vi "Amp_Lat_Finder.vi"(1 "ERP_vector":dbl[](array[numeric])) -> (0 "LDA_Parameter":dbl[][](array[numeric]))   [LabVIEW 2014]
uses:
  <vilib>/Analysis/baseanly.llb/Mean (DBL).vi
  <vilib>/Analysis/NI_AALBase.lvlib
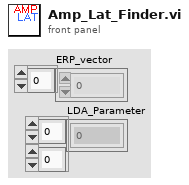
[diagram p1: front panel]
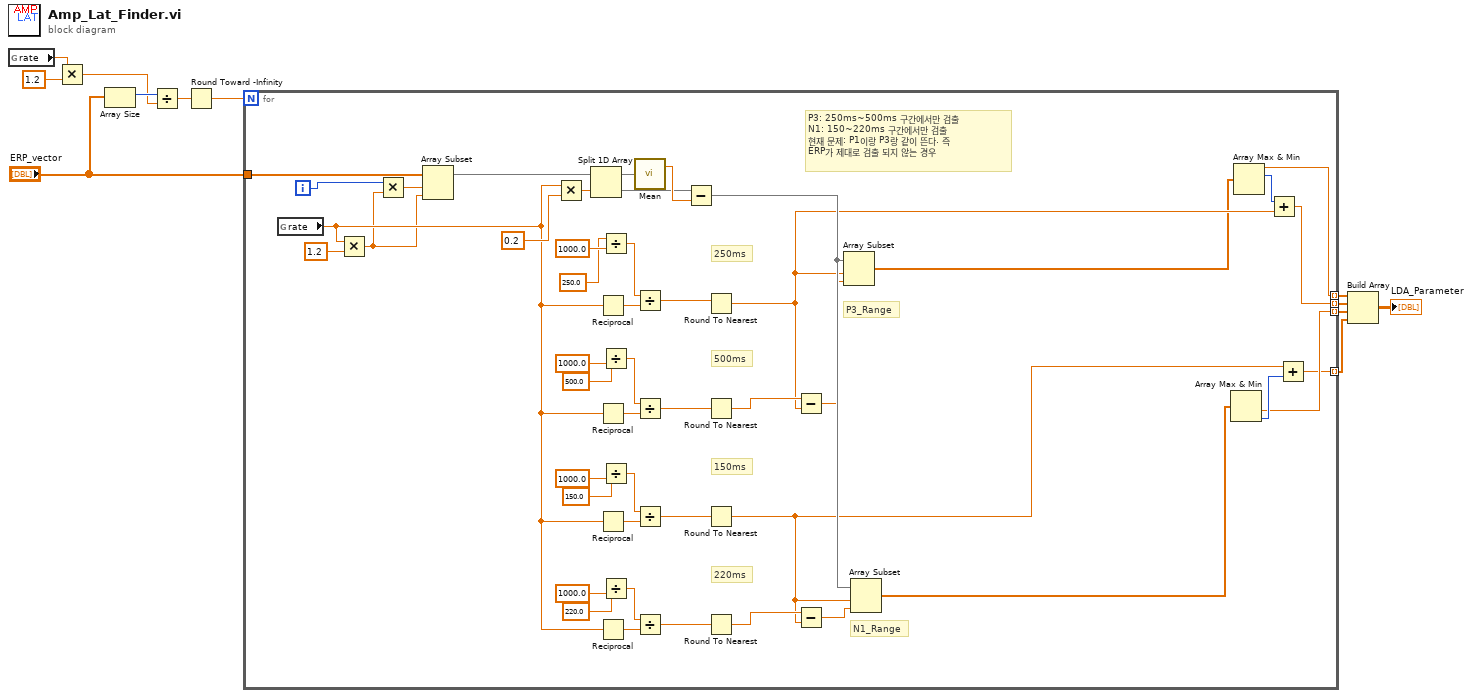
[diagram p0: block diagram]
diagram:
  n1 = global read "Control_Panel_정리.vi" "rate"() -> (w7:dbl)
  n2 = Multiply(x=w7, y=1.2) -> (x*y=w4:dbl)
  n3 = Array Size(array="ERP_vector") -> (size(s)=w5:i32)
  n4 = Divide(x=w5, y=w4) -> (x/y=w3:dbl)
  n5 = Round Toward -Infinity(1:w3) -> (0:w2:dbl)
  n6 = for {
    N: w2 -> [_]
    tunnel: "ERP_vector" -> [w25]
    tunnel: [w22] -> w12 mode=indexing
    tunnel: [w21] -> w11 mode=indexing
    tunnel: [w20] -> w10 mode=indexing
    tunnel: [w19] -> w9 mode=indexing
    i -> [w13]
    # "N1_Range"
    # "P3_Range"
    # "220ms"
    # "150ms"
    # "500ms"
    # "250ms"
    # "P3: 250ms~500ms 구간에서만 검출\nN1: 150~220ms 구간에서만 검출\n현재 문제: P1이랑 P3랑 같이 뜬다. 즉\nERP가 제대로 검출 되지 않는 경우"
    n7 = global read "Control_Panel_정리.vi" "rate"() -> (w18:dbl)
    n8 = Multiply(x=w18, y=1.2) -> (x*y=w14:dbl)
    n9 = Multiply(x=w13, y=w14) -> (x*y=w15:dbl)
    n10 = Array Subset(array=w25, index=w15, length=w14) -> (w16:dbl[])
    n11 = Multiply(x=w18, y=0.2) -> (x*y=w24:dbl)
    n12 = Split 1D Array(array=w16, index=w24) -> (first subarray=w59:dbl[], second subarray=w55:dbl[])
    n13 = Reciprocal(x=w18) -> (1/x=w54:dbl)
    n14 = Reciprocal(x=w18) -> (1/x=w53:dbl)
    n15 = Reciprocal(x=w18) -> (1/x=w52:dbl)
    n16 = Reciprocal(x=w18) -> (1/x=w51:dbl)
    n17 = Divide(x=250.0, y=1000.0) -> (x/y=w50:dbl)
    n18 = Divide(x=500.0, y=1000.0) -> (x/y=w49:dbl)
    n19 = Divide(x=150.0, y=1000.0) -> (x/y=w48:dbl)
    n20 = Divide(x=220.0, y=1000.0) -> (x/y=w47:dbl)
    n21 = call-poly <vilib>:"Mean.vi"("X"=w59) -> ("mean"=w58:dbl)  [unwired: 1 out]
    n22 = Divide(x=w50, y=w54) -> (x/y=w38:dbl)
    n23 = Divide(x=w49, y=w53) -> (x/y=w37:dbl)
    n24 = Divide(x=w48, y=w52) -> (x/y=w36:dbl)
    n25 = Divide(x=w47, y=w51) -> (x/y=w35:dbl)
    n26 = Subtract(x=w55, y=w58) -> (x-y=w32:dbl[])
    n27 = Round To Nearest(number=w38) -> (nearest integer value=w31:dbl)
    n28 = Round To Nearest(number=w37) -> (nearest integer value=w34:dbl)
    n29 = Round To Nearest(number=w36) -> (nearest integer value=w29:dbl)
    n30 = Round To Nearest(number=w35) -> (nearest integer value=w33:dbl)
    n31 = Subtract(x=w34, y=w31) -> (x-y=w30:dbl)
    n32 = Subtract(x=w33, y=w29) -> (x-y=w28:dbl)
    n33 = Array Subset(array=w32, index=w31, length=w30) -> (w27:dbl[])
    n34 = Array Subset(array=w32, index=w29, length=w28) -> (w26:dbl[])
    n35 = Array Max & Min(array=w26) -> (min value=w20:dbl, min index (indices)=w56:i32)  [unwired: 2 out]
    n36 = Array Max & Min(array=w27) -> (max value=w22:dbl, max index (indices)=w57:i32)  [unwired: 2 out]
    n37 = Add(x=w57, y=w31) -> (x+y=w21:dbl)
    n38 = Add(x=w29, y=w56) -> (x+y=w19:dbl)
  }
  n39 = Build Array(w12, w11, w10, w9) -> (→"LDA_Parameter":dbl[][])
